vi "Login Data.vi"() -> ()   [LabVIEW 2017]
panel:
  out "Login":bool
  out "Role Id":string
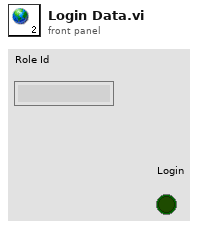
[diagram p1: front panel]
diagram:
